vi "Proj 2.vi"() -> ()   [LabVIEW 2018]
panel:
  in  "Slide":dbl(slide) scale=0.0..100.0
  out "Numeric 6":dbl
  out "Numeric 5":dbl
  in  "Numeric 4":dbl
  in  "Numeric 3":dbl
  in  "Numeric 2":dbl
  in  "Numeric":dbl
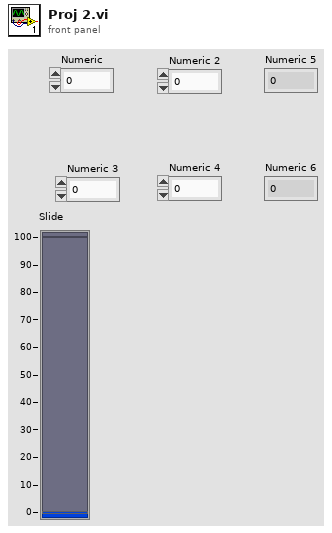
[diagram p1: front panel]
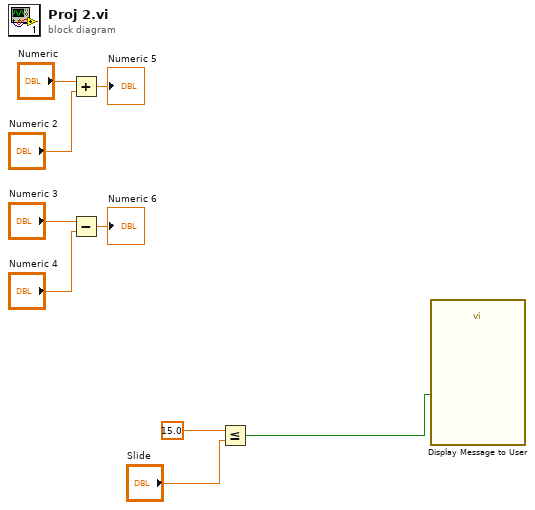
[diagram p0: block diagram]
diagram:
  n1 = Add(x="Numeric", y="Numeric 2") -> (x+y=→"Numeric 5":dbl)
  n2 = Subtract(x="Numeric 3", y="Numeric 4") -> (x-y=→"Numeric 6":dbl)
  n3 = Less Or Equal?(x=15.0, y="Slide") -> (x <= y?=w1:bool)
  n4 = call "Display Message to User"("Enable"=w1) -> ()  [unwired: 9 in, 2 out]
